vi "Complex QZ Decomposition.vi"(0 "A":T2, 5 "B":T2, 7 "decomposition type":i32(ring) items=["Generalized Hessenberg", "Generalized Schur"], 9 "order":T1 items=["No Reorder", "Real Ascending", "Real Descending", "Magnitude Ascending", "Magnitude Descending"]) -> (3 "Eigenvectors":T2, 4 "Q":T2, 6 "Z":T2, 8 "Alpha":cdb[](array[numeric]), 10 "Beta":cdb[](array[numeric]), 15 "error":i32)   [LabVIEW 2017, in "NI_AALPro.lvlib"]
doc: "Performs the QZ decomposition of a pair of square matrices. The data types you wire to the <B>A</B> and <B>B</B> inputs determine the polymorphic instance to use."
uses:
  <vilib>/Analysis/NI_AALPro.lvlib
  <vilib>/Analysis/Matrix/Datatypes/ComplexMatrix.ctl
  <vilib>/Analysis/7linalg.llb/Eigenvalue Order.ctl
  <vilib>/Analysis/Matrix/NI_Matrix.lvlib
  <resource>/lvanlys.dll
panel:
  # "QZ Decomposition"
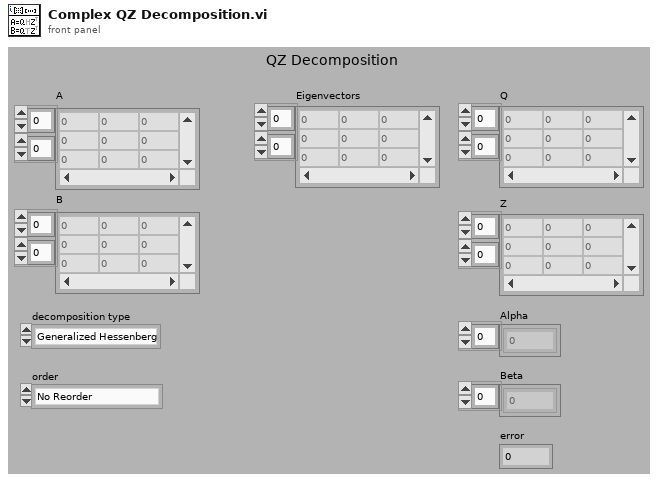
[diagram p1: front panel]
types:
  T1 = typedef "NI_AALPro.lvlib/Eigenvalue Order.ctl" = u16
  T2 = typedef "NI_Matrix.lvlib/ComplexMatrix.ctl" = cdb[][]
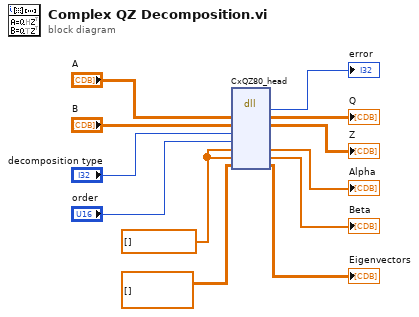
[diagram p0: block diagram]
diagram:
  w3 = cdb[] []
  n1 = dll-call lib="e:/builds/penguin/labview/branches/2017/dev/dist/resource/lvanlys.*" fn="CxQZ80_head"("A"="A", "B"="B", "type"="decomposition type", "orderOpt"="order", "output param"=w3, "output param"=w3, "Eigenvectors"=T2 []) -> (→"error":i32, "A"=→"Q":T2, "B"=→"Z":T2, "output param"=→"Alpha":cdb[], "output param"=→"Beta":cdb[], "Eigenvectors"=→"Eigenvectors":T2)  [unwired: 5 in, 2 out]
